vi "WaitForSpecificCommResponses.vi"(6 "Check period (msecs)":dbl=30.0, 8 "error in (no error)":errorcluster, 9 "Timeout (mSecs)":dbl=3000.0, 10 "WaitFor Keywords":string[](array[string]), 11 "VISA Refnum in":refnum<visa-resource-name>="COM30") -> (0 "error out":errorcluster, 1 "timeout":bool, 2 "Response":string, 3 "VISA Refnum out":refnum<visa-resource-name>, 4 "Keyword found index":i32, 5 "Elapsed secs":dbl)   [LabVIEW 2024]
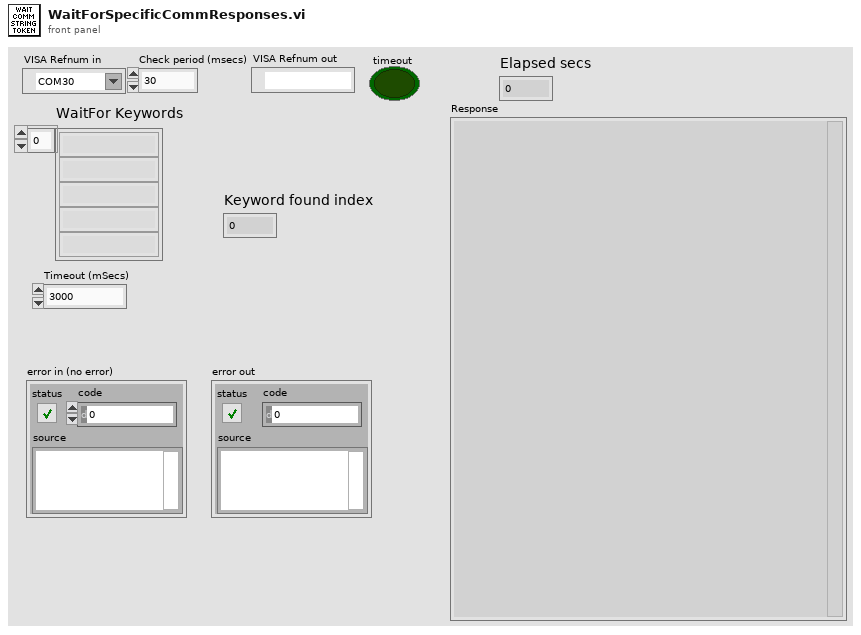
[diagram p1: front panel]
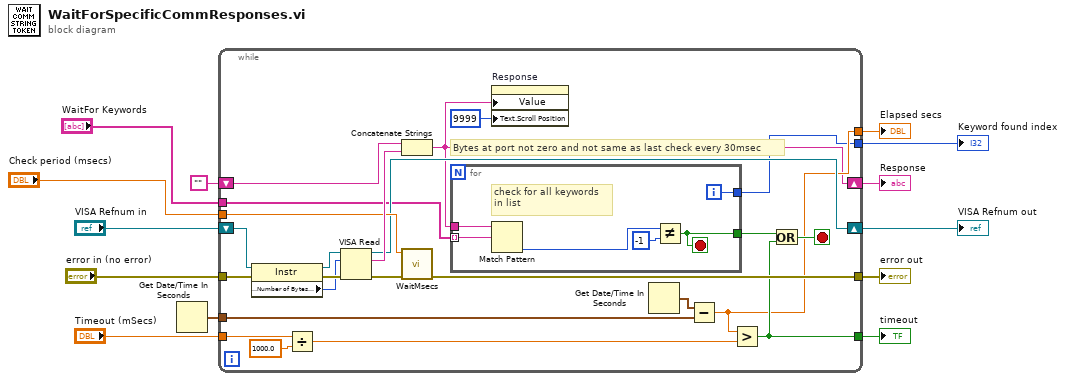
[diagram p0: block diagram]
diagram:
  n1 = Get Date/Time In Seconds() -> (seconds since 1Jan1904=w10:timestamp)
  n2 = while {
    shift-right: [w17] -> w9
    shift-left: "" -> [w34]
    tunnel: "error in (no error)" -> [w31]
    tunnel: [w29] -> w12
    tunnel: [w22] -> w4
    tunnel: "Timeout (mSecs)" -> [w27]
    tunnel: "Check period (msecs)" -> [w26]
    tunnel: w10 -> [w24]
    shift-right: [w20] -> w8
    shift-left: "VISA Refnum in" -> [w32]
    tunnel: [w19] -> w3
    tunnel: "WaitFor Keywords" -> [w18]
    tunnel: [w15] -> w1
    stop <- w28 stop-if-true
    # "Bytes at port not zero and not same as last check every 30msec"
    n3 = property class="Instr"(reference=w32, error in=w31) -> (reference out=w35:refnum<visa-resource-name>, error out=w37:errorcluster, "Serial Settings:Number of Bytes at Serial Port"=w36:u32)
    n4 = Divide(x=w27, y=1000.0) -> (x/y=w23:dbl)
    n5 = VISA Read(VISA resource name=w35, byte count=w36, error in (no error)=w37) -> (VISA resource name out=w20:refnum<visa-resource-name>, read buffer=w33:string, error out=w30:errorcluster)  [unwired: 1 out]
    n6 = Concatenate Strings(w34, w33) -> (w17:string)
    n7 = call "WaitMsecs.vi"("error in (no error)"=w30, "Wait Msecs"=w26) -> ("error out"=w29:errorcluster)  [unwired: 9 in]
    n8 = for {
      tunnel: w18 -> [w42] mode=indexing
      tunnel: w17 -> [w43]
      tunnel: [w39] -> w16
      tunnel: [w38] -> w15
      i -> [w38]
      stop <- w39 stop-if-true
      # "check for all keywords\nin list"
      n9 = Match Pattern(string=w43, regular expression=w42) -> (offset past match=w40:i32)  [unwired: 1 in, 3 out]
      n10 = Not Equal?(x=w40, y=-1) -> (x != y?=w39:bool)
    }
    n11 = property on="Response" class="Str"("Value"=w17, "Text.Scroll Position"=u32 9999) -> ()  [unwired: 2 in, 2 out]
    n12 = Get Date/Time In Seconds() -> (seconds since 1Jan1904=w25:timestamp)
    n13 = Subtract(x=w25, y=w24) -> (x-y=w19:dbl)
    n14 = Greater?(x=w19, y=w23) -> (0:w22:bool)
    n15 = Or(x=w16, y=w22) -> (x .or. y?=w28:bool)
  }
  "error out" <- w12
  "timeout" <- w4
  "VISA Refnum out" <- w8
  "Response" <- w9
  "Elapsed secs" <- w3
  "Keyword found index" <- w1
